vi "Stand Alone Cryogen.vi"() -> ()   [LabVIEW 2023, in "Level Meter.lvclass"]
uses:
  Level Meter/Level Meter.lvclass
  Level Meter/Cryogen Levels.ctl
panel:
  out "cryogenlvls":T1 min=-1.0 max=100.0 scale=0.0..100.0
  in  "endprogram":bool
  # "Reading and saving the cryogen levels."
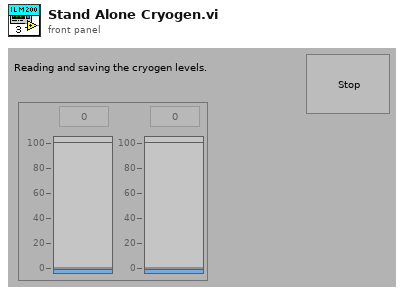
[diagram p1: front panel]
types:
  T1 = typedef "Level Meter.lvclass/Cryogen Levels.ctl" = dbl[]
  T2 = typedef "Readable.lvclass/X array.ctl" = T3[]
  T3 = typedef "Readable.lvclass/X.ctl" = dbl
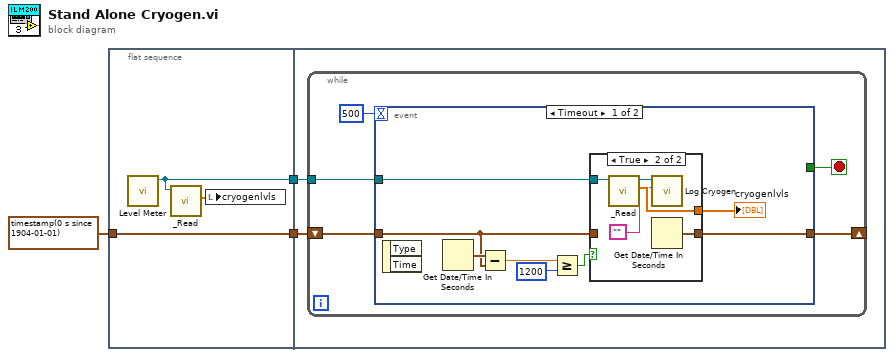
[diagram p0: block diagram]
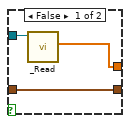
[diagram p2: hidden frame]
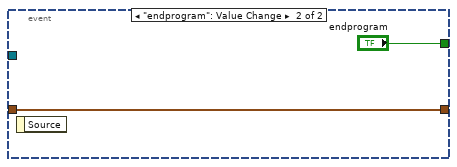
[diagram p3: hidden frame]
diagram:
  n1 = flat-sequence {
    tunnel: timestamp(0 s since 1904-01-01) ("seconds since 1Jan1904") -> [w6]
    tunnel: [w6] -> w2
    tunnel: [w5] -> w1
    tunnel: w2 -> [w8]
    tunnel: w1 -> [w7]
    frame #0 {
      n2 = call "Level Meter.vi"() -> ("Level Meter out"=w5:refnum<class "Level Meter.lvclass">)  [unwired: 10 in, 1 out]
      n3 = call-dynamic "_Read.vi"("Level Meter in"=w5) -> ("X array"=w4:T2)  [unwired: 8 in, 2 out]
      n4 = local write "cryogenlvls"(w4) -> ()
    }
    frame #1 {
      n5 = while {
        shift-right: [w13] -> _
        shift-left: w8 -> [w12]
        tunnel: w7 -> [w9]
        stop <- w11 stop-if-true
        n6 = event shown="[0] Timeout" {
          selector: _ -> [_ _]
          dyn-events: _ -> [_ _]
          timeout: 500 -> [_ _]
          tunnel: [w18 w30] -> w13
          tunnel: w12 -> [w17 w30]
          tunnel: [_ "endprogram"] -> w11
          tunnel: w9 -> [w14 _]
          event Timeout {
            n7 = event-data() -> ()  [unwired: 3 out]
            n8 = Get Date/Time In Seconds() -> (seconds since 1Jan1904=w21:timestamp)
            n9 = Subtract(x=w21, y=w17) -> (x-y=w20:dbl)
            n10 = Greater Or Equal?(x=w20, y=1200) -> (x >= y?=w19:bool)
            n11 = case shown="True" w19 {
              tunnel: [w24 w29] -> w18
              tunnel: w17 -> [w24 _]
              tunnel: [w23 w27] -> w15
              tunnel: w14 -> [w22 w28]
              frame False {
                n12 = call-dynamic "_Read.vi"("Level Meter in"=w22) -> ("X array"=w23:T2)  [unwired: 8 in, 2 out]
              }
              frame True {
                n13 = call-dynamic "_Read.vi"("Level Meter in"=w28) -> ("X array"=w27:T2, "Level Meter out"=w26:refnum<class "Level Meter.lvclass">)  [unwired: 8 in, 1 out]
                n14 = call-dynamic "Log Cryogen.vi"("Status string"="", "Level Meter in"=w26) -> ()  [unwired: 8 in, 2 out]
                n15 = Get Date/Time In Seconds() -> (seconds since 1Jan1904=w29:timestamp)
              }
            }
            "cryogenlvls" <- w15
          }
          event "endprogram": Value Change {
            n16 = event-data() -> ()  [unwired: 2 out]
          }
        }
      }
    }
  }
